vi "ReadTrajectoryCalibFile.vi"(8 "error in (no error)":errorcluster, 11 "Spec_Calib_file in":path) -> (0 "error out":errorcluster, 3 "Cluster":T1)   [LabVIEW 2013]
uses:
  CalibrationCluster.ctl
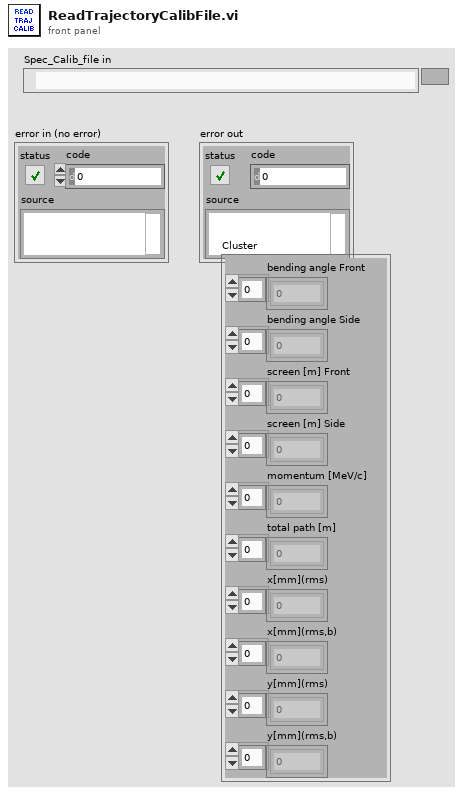
[diagram p1: front panel]
types:
  T1 = typedef "CalibrationCluster.ctl" = cluster{"bending angle Front":dbl[], "bending angle Side":dbl[], "screen [m] Front":dbl[], "screen [m] Side":dbl[], "momentum [MeV/c]":dbl[], "total path [m]":dbl[], "x[mm](rms)":dbl[], "x[mm](rms,b)":dbl[], "y[mm](rms)":dbl[], "y[mm](rms,b)":dbl[]}
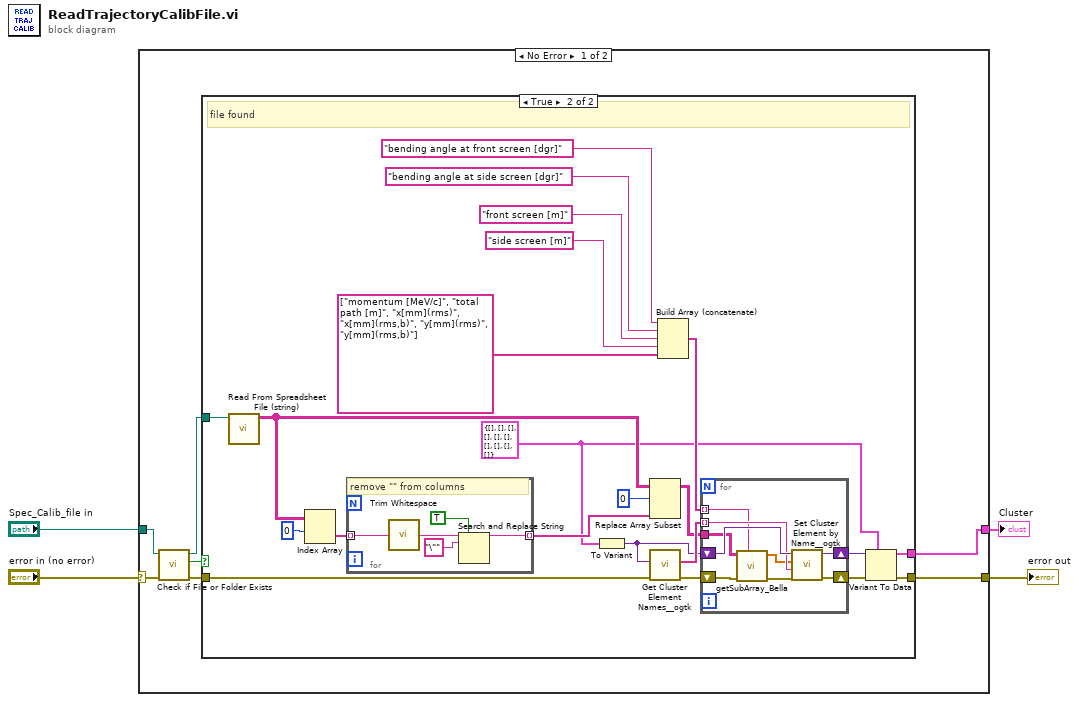
[diagram p0: block diagram]
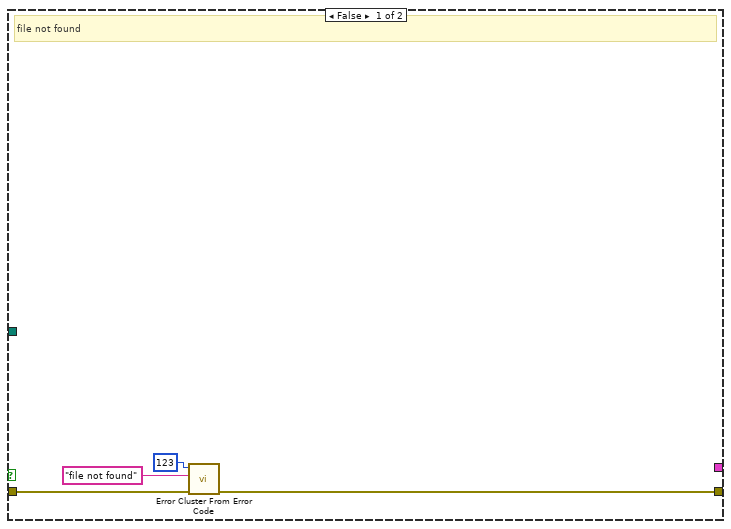
[diagram p2: hidden frame]
diagram:
  n1 = case shown="No Error" "error in (no error)" {
    selector: "error in (no error)" -> [w6 w52]
    tunnel: [w11 w52] -> w4
    tunnel: [w10 _] -> w1
    tunnel: "Spec_Calib_file in" -> [w7 _]
    frame No Error {
      n2 = call "Check if File or Folder Exists.vi"("error in (no error)"=w6, "path"=w7) -> ("error out"=w9:errorcluster, "file or folder exists?"=w5:bool, "dup path"=w8:path)  [unwired: 7 in]
      n3 = case shown="True" w5 {
        tunnel: [w12 w37] -> w11
        tunnel: [_ w34] -> w10
        tunnel: w9 -> [w13 w28]
        tunnel: w8 -> [_ w27]
        frame False {
          # "file not found"
          n4 = call "Error Cluster From Error Code.vi"("error in (no error)"=w13, "error message (\"\")"="file not found" ("source"), "error code (0)"=123 ("code")) -> ("error out"=w12:errorcluster)  [unwired: 6 in]
        }
        frame True {
          w20 = T1 {"bending angle Front"=[], "bending angle Side"=[], "screen [m] Front"=[], "screen [m] Side"=[], "momentum [MeV/c]"=[], "total path [m]"=[], "x[mm](rms)"=[], "x[mm](rms,b)"=[], "y[mm](rms)"=[], "y[mm](rms,b)"=[]} ("Cluster")
          # "file found"
          n5 = call "Read From Spreadsheet File (string).vi"("file path (dialog if empty)"=w27) -> ("all rows"=w24:string[][])  [unwired: 6 in, 4 out]
          n6 = Index Array(array=w24, index (row)=0) -> (element=w25:string[])  [unwired: 1 in]
          n7 = for {
            tunnel: w25 -> [w42] mode=indexing
            tunnel: [w39] -> w22 mode=indexing
            # "remove \"\" from columns"
            n8 = call "Trim Whitespace.vi"("string"=w42) -> ("trimmed string"=w41:string)  [unwired: 1 in]
            n9 = Search and Replace String(replace all?=TRUE ("replace all? (F)"), input string=w41, search string="\"") -> (result string=w39:string)  [unwired: 5 in, 3 out]
          }
          n10 = To Variant(anything=w20) -> (Variant=w32:variant)
          n11 = Replace Array Subset(array=w24, new element=w22, index (row)=0) -> (w21:string[][])  [unwired: 1 in]
          n12 = call "Get Cluster Element Names__ogtk.vi"("error in (no error)"=w28, "Cluster"=w32) -> ("error out"=w35:errorcluster, "Element Names"=w33:string[])  [unwired: 8 in]
          n13 = Build Array (concatenate)("bending angle at front screen [dgr]" ("element"), "bending angle at side screen [dgr]" ("element"), "front screen [m]" ("element"), "side screen [m]" ("element"), string[] ["momentum [MeV/c]", "total path [m]", "x[mm](rms)", "x[mm](rms,b)", "y[mm](rms)", "y[mm](rms,b)"]) -> (w30:string[])
          n14 = for {
            tunnel: w30 -> [w47] mode=indexing
            tunnel: w21 -> [w46]
            shift-right: [w50] -> w31
            shift-left: w32 -> [w51]
            tunnel: w33 -> [w49] mode=indexing
            shift-right: [w48] -> w36
            shift-left: w35 -> [w45]
            n15 = call "getSubArray_Bella.vi"("element"=w47, "error in (no error)"=w45, "Array IN"=w46) -> ("error out"=w43:errorcluster, "Array out"=w44:dbl[])  [unwired: 7 in]
            n16 = call "Set Cluster Element by Name__ogtk.vi"("error in (no error)"=w43, "Element Name (\"\": New Element Data Name)"=w49, "New Element Value"=w44, "Cluster"=w51) -> ("error out"=w48:errorcluster, "VCluster out"=w50:variant)  [unwired: 5 in, 1 out]
          }
          n17 = Variant To Data(error in=w36, type=w20, Variant=w31) -> (data=w34:T1, error out=w37:errorcluster)
        }
      }
    }
    frame Error {
    }
  }
  "error out" <- w4
  "Cluster" <- w1
